vi "getAcquisitionReady.vi"(6 "Delay between send and receive [ms]":i32=100, 8 "error in (no error)":errorcluster, 11 "CCD in":refnum<class "CCD.lvclass">) -> (0 "error out":errorcluster, 2 "ready":bool, 3 "CCD out":refnum<class "CCD.lvclass">)   [LabVIEW 2020, in "horiba.lvlib" / "CCD.lvclass"]
doc: "Queries the CCD for readiness for acquisition."
uses:
  CCD.lvclass
  AcquisitionReady.ctl
  20f7d3bd-08ac-4524-9bed-df36c1da25a0.vi
  a21955fc-e3a0-4e36-8495-41f1bfac7860.vi
  <vilib>/JDP Science/JSONtext/Variant to JSON Text.vi
  <vilib>/JDP Science/JSONtext/Set Item.vi
  <vilib>/JDP Science/JSONtext/JSON text to Variant.vi
  <vilib>/JDP Science/JSONtext/LVClass Serializer/JSONtext LVClass Serializer.lvclass
  GenericDevice/GenericDevice.lvclass
panel:
  # "Connector Pane"
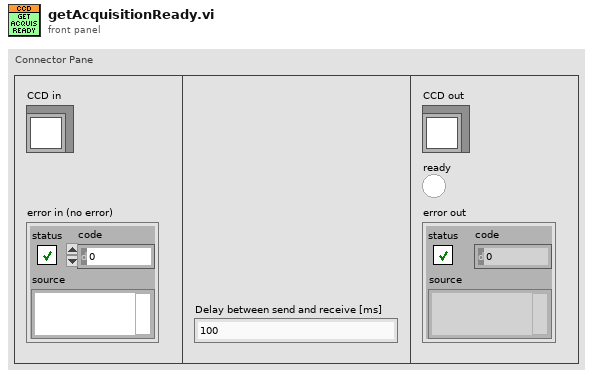
[diagram p1: front panel]
types:
  T1 = typedef "horiba.lvlib/CCD.lvclass/AcquisitionReady.ctl" = cluster{"ready":bool}
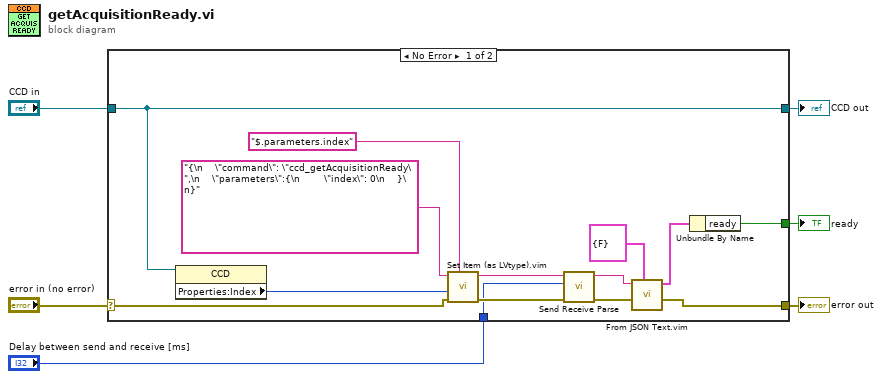
[diagram p0: block diagram]
diagram:
  n1 = case shown="No Error" "error in (no error)" {
    selector: "error in (no error)" -> [w16 w22]
    tunnel: [w15 w22] -> w5
    tunnel: [w18 w21] -> w3
    tunnel: "CCD in" -> [w18 w21]
    tunnel: [w10 _] -> w2
    tunnel: "Delay between send and receive [ms]" -> [w8 _]
    frame No Error {
      n2 = property on="Property Node" class="CCD"(reference=w18) -> ("Properties:Index"=w17:i32)  [unwired: 1 in, 2 out]
      n3 = call "Set Item (as LVtype).vim"("$Path or Item Name"="$.parameters.index", "error in (no error)"=w16, "Anything"=w17, "JSON"="{\n    \"command\": \"ccd_getAcquisitionReady\",\n    \"parameters\":{\n        \"index\": 0\n    }\n}") -> ("error out"=w13:errorcluster, "<JSON>"=w7:string)  [unwired: 4 in, 1 out]
      n4 = call "Send Receive Parse.vi"("error in"=w13, "Delay between send and receive [ms]"=w8, "<JSON>"=w7) -> ("error out"=w12:errorcluster, "results-JSON string"=w14:string)  [unwired: 6 in, 1 out]
      n5 = call "From JSON Text.vim"("Data Type and Default Value"=T1 {"ready"=FALSE} ("ccd acquisition ready?"), "error in (no error)"=w12, "JSON"=w14) -> ("error out"=w15:errorcluster, "Data out"=w11:T1)  [unwired: 7 in]
      n6 = Unbundle By Name(w11) -> ("ready"=w10:bool)
    }
    frame Error {
    }
  }
  "error out" <- w5
  "CCD out" <- w3
  "ready" <- w2
